vi "destroyEvents.vi"(8 "error in (no error)":errorcluster, 11 "TCPComEvents in":refnum<class "TCPComEvents.lvclass">) -> (0 "error out":errorcluster, 3 "TCPComEvents out":refnum<class "TCPComEvents.lvclass">)   [LabVIEW 2016, in "TCPComEvents.lvclass"]
uses:
  TCPComEvents.lvclass
  TCPComEvents.lvclass/TCPComEvents.ctl
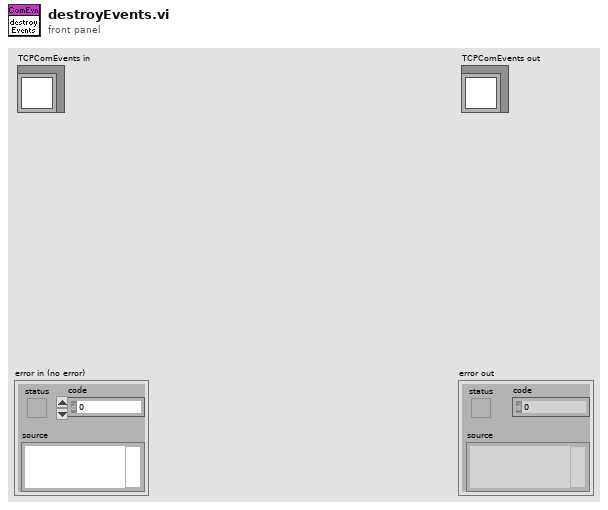
[diagram p1: front panel]
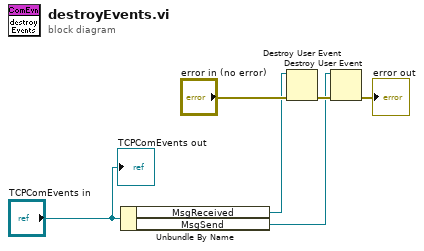
[diagram p0: block diagram]
diagram:
  n1 = Unbundle By Name("TCPComEvents in") -> ("MsgReceived"=w5:refnum<user-event>, "MsgSend"=w1:refnum<user-event>)
  n2 = Destroy User Event(user event=w5, error in="error in (no error)") -> (error out=w3:errorcluster)
  n3 = Destroy User Event(user event=w1, error in=w3) -> (error out=→"error out":errorcluster)
  "TCPComEvents out" <- "TCPComEvents in"
